vi "Read Assert Only_.vi"(8 "error in (no error)":errorcluster, 11 "Assert":refnum<class "Assert.lvclass">) -> (0 "error out":errorcluster, 2 "Assert Only?":bool, 3 "Assert":refnum<class "Assert.lvclass">)   [LabVIEW 2013, in "Caraya.lvlib" / "Assert.lvclass"]
uses:
  Assert/Assert.lvclass
  Assert/Assert.lvclass/Assert.ctl
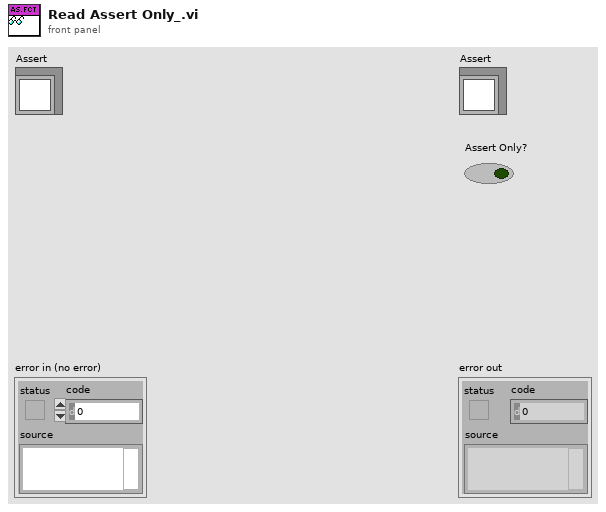
[diagram p1: front panel]
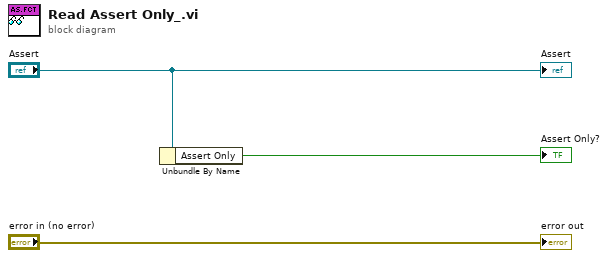
[diagram p0: block diagram]
diagram:
  n1 = Unbundle By Name("Assert") -> ("Assert Only"=→"Assert Only?":bool)
  "error out" <- "error in (no error)"
  "Assert" <- "Assert"
